vi "Read Table.vi"(0 "Display State In":T1, 5 "Type of Anything":variant, 9 "Container State":T6, 11 "error in (no error)":errorcluster) -> (4 "Display State Out":T1, 6 "Value":variant, 15 "error out":errorcluster)   [LabVIEW 2020, in "KTable.xctl"]
uses:
  KTable.xctl
  <vilib>/_xctls/Container State.ctl
  State.ctl
  ColumnSpec.ctl
  ColumnType.ctl
  Table Properties.ctl
  Events.ctl
  Event Data.ctl
  Event Type.ctl
  Array Manipulation VIs/Array-Dimensions (2D string).vi
  <vilib>/_xctls/XControlSupport.lvlib
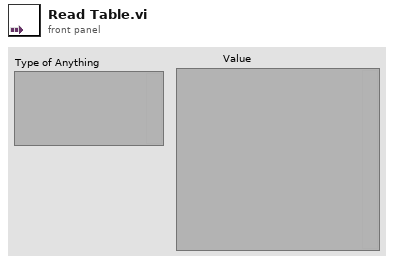
[diagram p1: front panel]
types:
  T1 = typedef "KTable.xctl/State.ctl" = cluster{"Columns":T2[], "Listbox":refnum<vi>, "Default row":string[], "Properties":T4, "Events":T5, "Locked":bool[][], "Size":cluster{"Rows":i32, "Columns":i32}, "rings":i32[][], "DefColors":u32[]}
  T2 = typedef "KTable.xctl/ColumnSpec.ctl" = cluster{"Name":string, "Type":T3, "Width":i32, "Strings":string[], "Position":enum16{"Left", "Center", "Right"}, "locked":bool, "cds":cluster{"Strings":string[]}[][], "Hide NaN":bool}
  T3 = typedef "KTable.xctl/ColumnType.ctl" = enum16{"String", "Enum", "Int", "Double", "Boolean", "Ring", "Formula", "Color"}
  T4 = typedef "KTable.xctl/Table Properties.ctl" = cluster{"Vertical scrollbar":bool, "User add/delete":bool, "Max rows":i32, "Row headers":bool}
  T5 = typedef "KTable.xctl/Events.ctl" = cluster{"Items Changed":refnum<user-event>}
  T6 = typedef "XControlSupport.lvlib/Container State.ctl" = cluster{"Indicator?":bool, "Run Mode?":bool, " Refnum":refnum<vi>}
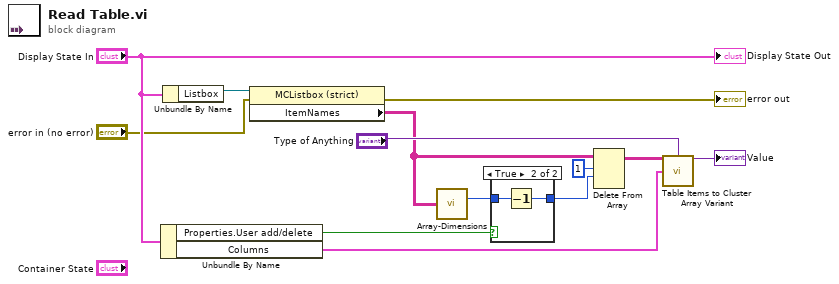
[diagram p0: block diagram]
diagram:
  n1 = Unbundle By Name("Display State In") -> ("Properties.User add/delete"=w1:bool, "Columns"=w12:T2[])
  n2 = Unbundle By Name("Display State In") -> ("Listbox"=w13:refnum<vi>)
  n3 = property class="MCListbox (strict)"(reference=w13, error in="error in (no error)") -> (error out=→"error out":errorcluster, "ItemNames"=w4:string[][])  [unwired: 1 out]
  n4 = call-poly "Array-Dimensions.vi"("2D Array"=w4) -> ("# rows"=w3:i32)  [unwired: 13 in, 1 out]
  n5 = case shown="True" w1 {
    tunnel: w3 -> [w14 w16]
    tunnel: [w14 w15] -> w2
    frame False {
    }
    frame True {
      n6 = Decrement(x=w16) -> (x-1=w15:i32)
    }
  }
  n7 = Delete From Array(array=w4, length=1, index (row)=w2) -> (array with subset deleted=w5:string[][])  [unwired: 1 in, 1 out]
  n8 = call "Table Items to Cluster Array Variant.vi"("Table Items"=w5, "Type of Anything"="Type of Anything", "Columns"=w12) -> ("Anything"=→"Value":variant)  [unwired: 11 in, 1 out]
  "Display State Out" <- "Display State In"
